vi "Set Fast File Format.vi"(8 "error in (no error)":errorcluster, 10 "Enable Fast File Format":bool, 11 "NI_AB_API_EXE_Extensions in":refnum<class "NI_AB_API_EXE_Extensions.lvclass">) -> (0 "error out":errorcluster, 3 "NI_AB_API_EXE_Extensions out":refnum<class "NI_AB_API_EXE_Extensions.lvclass">)   [LabVIEW 2021, in "NI_AB_API_EXE_Extensions.lvclass"]
uses:
  NI_AB_API_EXE_Extensions.lvclass
  NI_AB_API_EXE_Extensions.lvclass/NI_AB_API_EXE_Extensions.ctl
  <vilib>/AppBuilder/AB_Classes/TargetFile/AB_Targetfile.lvclass
  <vilib>/AppBuilder/AB_API/Build/NI_AB_API_Build.lvclass
  <vilib>/AppBuilder/AB_Classes/EXE/AB_EXE.lvclass
  C:/Program Files/National Instruments/LabVIEW 2021/vi.lib/AppBuilder/AB_API/EXE/NI_AB_API_EXE.lvclass
  C:/Program Files/National Instruments/LabVIEW 2021/vi.lib/AppBuilder/AB_API/Application/NI_AB_API_Application.lvclass
  C:/Program Files/National Instruments/LabVIEW 2021/vi.lib/AppBuilder/AB_API/Targetfile/NI_AB_API_Targetfile.lvclass
  C:/Program Files/National Instruments/LabVIEW 2021/vi.lib/AppBuilder/AB_API/Build/NI_AB_API_Build.lvclass
  C:/Program Files/National Instruments/LabVIEW 2021/vi.lib/AppBuilder/AB_Classes/Application/AB_Application.lvclass
  C:/Program Files/National Instruments/LabVIEW 2021/vi.lib/AppBuilder/AB_Classes/TargetFile/AB_Targetfile.lvclass
  C:/Program Files/National Instruments/LabVIEW 2021/vi.lib/AppBuilder/AB_Classes/Build/AB_Build.lvclass
  C:/Program Files/National Instruments/LabVIEW 2021/vi.lib/AppBuilder/AB_Classes/EXE/AB_EXE.lvclass
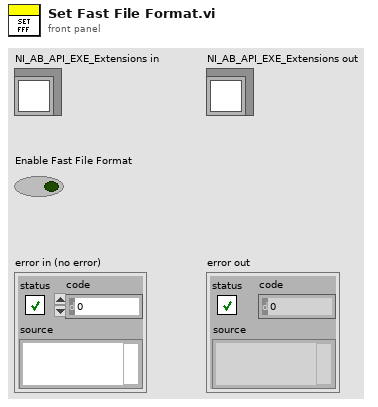
[diagram p1: front panel]
types:
  T1 = typedef "AB_Targetfile.ctl" = cluster{"targetfileName":string, "targetfileGUID":string, "enableDebugging":bool, "versionInfo":cluster{"productName":string, "legalCopyright":string, "companyName":string, "internalName":string, "fileDescription":string}, "eng_consolidatedTypeInfo":string, "fastFileFormat":bool, "eng_LEIFBuildData":u32, "versionIndependent":bool}
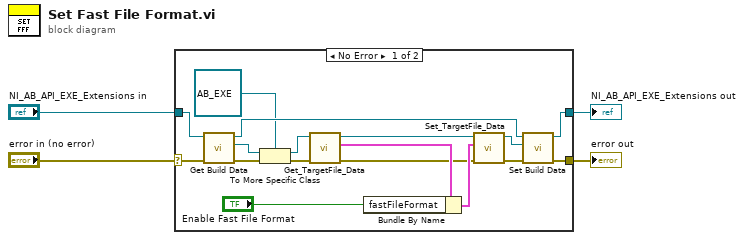
[diagram p0: block diagram]
diagram:
  n1 = case shown="No Error" "error in (no error)" {
    selector: "error in (no error)" -> [w8 w23]
    tunnel: [w7 w23] -> w3
    tunnel: [w9 w22] -> w1
    tunnel: "NI_AB_API_EXE_Extensions in" -> [w10 w22]
    frame No Error {
      n2 = call <vilib>:"Get Build Data.vi"("error in (no error)"=w8, "NI_AB_API_Build in"=w10) -> ("error out"=w15:errorcluster, "AB_Build.lvclass"=w17:refnum<class "AB_Build.lvclass">, "NI_AB_API_Build in"=w18:refnum<class "NI_AB_API_EXE_Extensions.lvclass">)  [unwired: 7 in]
      n3 = To More Specific Class(target class=refnum<class "AB_EXE.lvclass"> refnum ("AB_EXE.lvclass"), reference=w17, error in=w15) -> (specific class reference=w16:refnum<class "AB_EXE.lvclass">, error out=w13:errorcluster)
      n4 = call <vilib>:"Get_TargetFile_Data.vi"("error in (no error)"=w13, "AB_Targetfile in"=w16) -> ("error out"=w12:errorcluster, "data"=w20:T1, "AB_Targetfile out"=w21:refnum<class "AB_EXE.lvclass">)  [unwired: 7 in]
      n5 = Bundle By Name(cluster=w20, "fastFileFormat"="Enable Fast File Format") -> (w19:T1)
      n6 = call <vilib>:"Set_TargetFile_Data.vi"("error in (no error)"=w12, "data"=w19, "AB_Targetfile in"=w21) -> ("error out"=w11:errorcluster, "AB_Targetfile out"=w14:refnum<class "AB_EXE.lvclass">)  [unwired: 7 in]
      n7 = call <vilib>:"Set Build Data.vi"("error in (no error)"=w11, "AB_Build.lvclass"=w14, "NI_AB_API_Build in"=w18) -> ("error out"=w7:errorcluster, "NI_AB_API_Build in"=w9:refnum<class "NI_AB_API_EXE_Extensions.lvclass">)  [unwired: 7 in]
    }
    frame Error {
    }
  }
  "error out" <- w3
  "NI_AB_API_EXE_Extensions out" <- w1
